vi "DailyPatchBranchName.vi"() -> (3 "DailyPatchBranchName":string)   [LabVIEW 2017]
doc: "lvAPT-User-Libraries 2022.4.27.213228\nYAO - lvAPT\nCopyright (c) 2022, lvAPT"
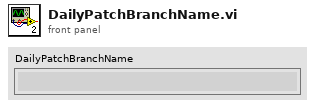
[diagram p1: front panel]
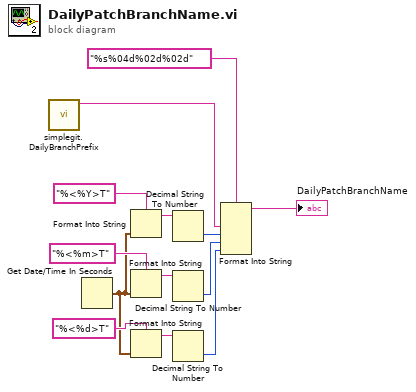
[diagram p0: block diagram]
diagram:
  n1 = call "simplegit.DailyBranchPrefix.vi"() -> ("value"=w1:string)  [unwired: 11 in]
  n2 = Get Date/Time In Seconds() -> (seconds since 1Jan1904=w2:timestamp)
  n3 = Format Into String(format string="%<%Y>T", w2) -> (resulting string=w3:string)  [unwired: 2 in, 1 out]
  n4 = Format Into String(format string="%<%m>T", w2) -> (resulting string=w4:string)  [unwired: 2 in, 1 out]
  n5 = Format Into String(format string="%<%d>T", w2) -> (resulting string=w5:string)  [unwired: 2 in, 1 out]
  n6 = Decimal String To Number(string=w3) -> (number=w10:i32)  [unwired: 2 in, 1 out]
  n7 = Decimal String To Number(string=w4) -> (number=w11:i32)  [unwired: 2 in, 1 out]
  n8 = Decimal String To Number(string=w5) -> (number=w12:i32)  [unwired: 2 in, 1 out]
  n9 = Format Into String(format string="%s%04d%02d%02d", w1, w10, w11, w12) -> (resulting string=→"DailyPatchBranchName":string)  [unwired: 2 in, 1 out]
